vi "AddTAFMenu.vi"(8 "ErrorIn":errorcluster, 10 "MenuIn":T1[](array[typedef]), 11 "DemoApplicationIn":refnum<class "DemoApplication.lvclass">) -> (0 "ErrorOut":errorcluster, 2 "MenuOut":T1[](array[typedef]), 3 "DemoApplicationOut":refnum<class "DemoApplication.lvclass">)   [LabVIEW 2021, in "DemoApplication.lvclass"]
uses:
  DemoApplication.lvclass
  .Externals/Library_TAF_ApplicationFramework/MasterGUI/MenuItem.ctl
  .Externals/Interface_TAF_ITAFObject/ITAFObject/ITAFObject.lvclass
  fc2f2e73-5f71-428f-9099-5e7628a6c5e6.vi
  .Externals/Library_TAF_ApplicationFramework/Application/Application_GetInstance.vi
  <vilib>/Utility/LVClass/Get LV Class Name.vi
  .Externals/Interface_TAF_IApplicationConfiguration/IApplicationConfiguration/IApplicationConfiguration.lvclass
  .Externals/Library_TAF_ApplicationFramework/MasterGUI/MasterGUI.lvclass
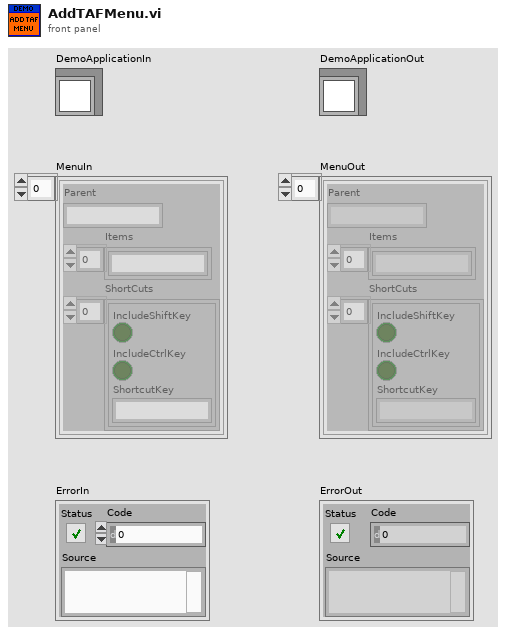
[diagram p1: front panel]
types:
  T1 = typedef "MasterGUI.lvclass/MenuItem.ctl" = cluster{"Parent":string, "Items":string[], "ShortCuts":cluster{"IncludeShiftKey":bool, "IncludeCtrlKey":bool, "ShortcutKey":string}[]}
  T2 = cluster{"IncludeShiftKey":bool, "IncludeCtrlKey":bool, "ShortcutKey":string}[]
  T3 = typedef "DemoApplication.lvclass/ObjectAttributes.ctl" = cluster{"Interfaces":cluster{"Authorizer":refnum<class "IAuthorization.lvclass">, "TextViewer":refnum<class "ITAFTextViewer.lvclass">, "ApplicationConfiguration":refnum<class "IApplicationConfiguration.lvclass">, "Tracer":refnum<class "IFrontPanel.lvclass">}, "Persistent":cluster{"MenuEnables":cluster{"MenuTag":string, "MenuExpression":string}[], "TextDockSubPanelName":string}}
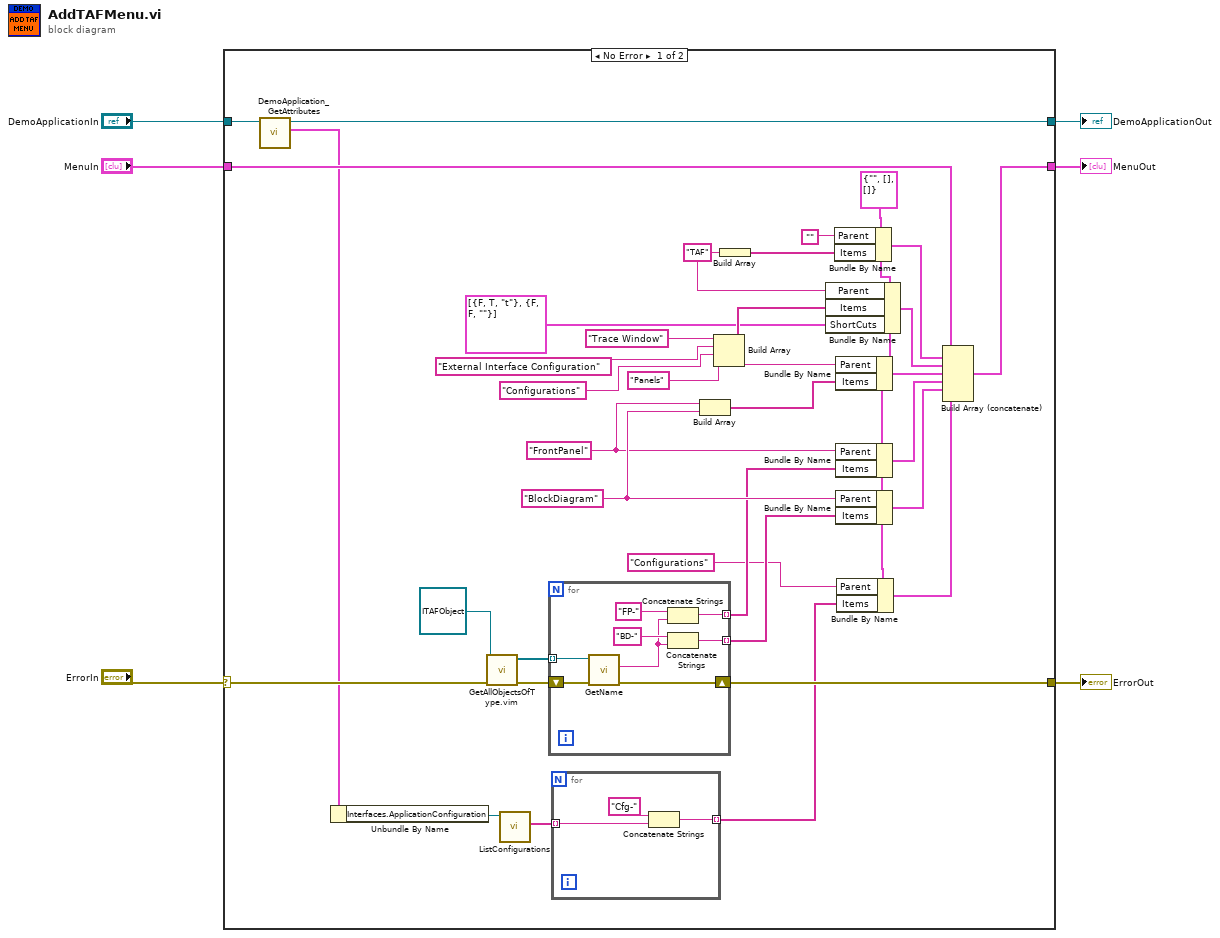
[diagram p0: block diagram]
diagram:
  n1 = case shown="No Error" "ErrorIn" {
    selector: "ErrorIn" -> [w39 w55]
    tunnel: [w41 w55] -> w6
    tunnel: [w38 w53] -> w4
    tunnel: [w15 w54] -> w2
    tunnel: "DemoApplicationIn" -> [w27 w54]
    tunnel: "MenuIn" -> [w26 w53]
    frame No Error {
      w22 = "TAF" ("Parent")
      w20 = "Panels" ("Parent")
      w33 = "BlockDiagram" ("Parent")
      w32 = "FrontPanel" ("Parent")
      w11 = T1 {"Parent"="", "Items"=[], "ShortCuts"=[]} ("MenuTree")
      n2 = call "DemoApplication_GetAttributes.vi"("ReferenceIn"=w27) -> ("Data"=w14:T3, "ReferenceOut"=w15:refnum<class "DemoApplication.lvclass">)  [unwired: 7 in, 2 out]
      n3 = Unbundle By Name(w14) -> ("Interfaces.ApplicationConfiguration"=w13:refnum<class "IApplicationConfiguration.lvclass">)
      n4 = call "GetAllObjectsOfType.vim"("ErrorIn"=w39, "ObjectType"=refnum<class "ITAFObject.lvclass"> refnum ("NamedCreator")) -> ("ErrorOut"=w40:errorcluster, "ObjectsOut"=w31:refnum<class "ITAFObject.lvclass">[])  [unwired: 8 in]
      n5 = call-dynamic "ListConfigurations.vi"("ObjectIn"=w13) -> ("Identification"=w12:string[])  [unwired: 8 in, 2 out]
      n6 = for {
        tunnel: w31 -> [w50] mode=indexing
        shift-right: [w51] -> w41
        shift-left: w40 -> [w52]
        tunnel: [w47] -> w29 mode=indexing
        tunnel: [w46] -> w28 mode=indexing
        n7 = call-dynamic "GetName.vi"("ErrorIn"=w52, "ObjectIn"=w50) -> ("ErrorOut"=w51:errorcluster, "Name"=w45:string)  [unwired: 7 in, 1 out]
        n8 = Concatenate Strings("FP-" ("string"), w45) -> (w46:string)
        n9 = Concatenate Strings("BD-" ("string"), w45) -> (w47:string)
      }
      n10 = for {
        tunnel: w12 -> [w44] mode=indexing
        tunnel: [w42] -> w9 mode=indexing
        n11 = Concatenate Strings("Cfg-" ("string"), w44) -> (w42:string)
      }
      n12 = Build Array(w32, w33) -> (w34:string[])
      n13 = Build Array("Trace Window" ("Parent"), "External Interface Configuration" ("Parent"), "Configurations" ("Parent"), w20) -> (w19:string[])
      n14 = Build Array(w22) -> (w24:string[])
      n15 = Bundle By Name(cluster=w11, "Parent"=w22, "Items"=w19, "ShortCuts"=T2 [{"IncludeShiftKey"=FALSE, "IncludeCtrlKey"=TRUE, "ShortcutKey"="t"}, {"IncludeShiftKey"=FALSE, "IncludeCtrlKey"=FALSE, "ShortcutKey"=""}]) -> (w37:T1)
      n16 = Bundle By Name(cluster=w11, "Parent"="", "Items"=w24) -> (w23:T1)
      n17 = Bundle By Name(cluster=w11, "Parent"=w20, "Items"=w34) -> (w35:T1)
      n18 = Bundle By Name(cluster=w11, "Parent"=w32, "Items"=w28) -> (w36:T1)
      n19 = Bundle By Name(cluster=w11, "Parent"=w33, "Items"=w29) -> (w17:T1)
      n20 = Bundle By Name(cluster=w11, "Parent"="Configurations", "Items"=w9) -> (w8:T1)
      n21 = Build Array (concatenate)(w26, w23, w37, w35, w36, w17, w8) -> (w38:T1[])
    }
    frame Error {
    }
  }
  "DemoApplicationOut" <- w2
  "ErrorOut" <- w6
  "MenuOut" <- w4
